vi "Orientation measurements standalone.vi"() -> ()   [LabVIEW 2016]
uses:
  <vilib>/rvi/interface/nirviReadWriteControl/nirviReadWriteControl.xnode
  FPGA Bitfiles/FPGAIMU_FPGATarget_FPGAIMURead_c-b2E2IVPMQ.lvbitx
  <vilib>/rvi/errors/niLvFpgaMergeErrorWithErrorCode.vi
  <vilib>/rvi/errors/niLvFpgaAdjustHostInterfaceError.vi
panel:
  out "Number of misses":i16
  out "Time to read start bit":u32
  out "Time to read data bits":u32
  out "Time to read 1 char":u32
  in  "ThirdTune":u32
  in  "SecondTune":u32=5
  in  "FirstTune":u32
  out "Fifo full?":bool
  in  "Bytes to Read":u32=38
  out "Output":cluster{dbl, dbl, bool}
  out "Error out":errorcluster
  in  "Stop":bool
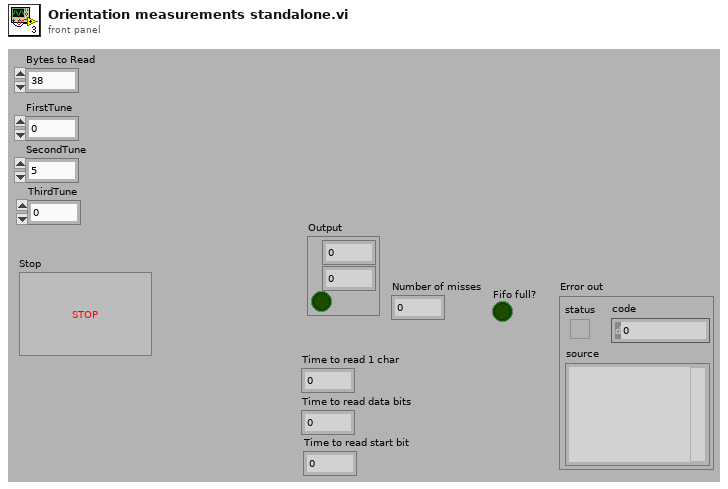
[diagram p1: front panel]
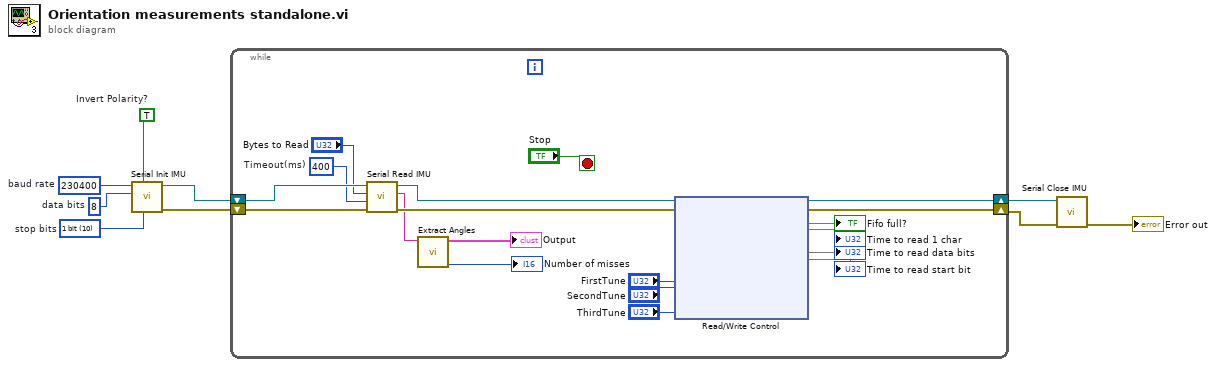
[diagram p0: block diagram]
diagram:
  w9 = u16 10 items=["1 bit"=10, "1.5 bits"=15, "2 bits"=20]  # stop bits
  w8 = 8  # data bits
  w6 = TRUE  # Invert Polarity?
  w7 = u32 230400  # baud rate
  n1 = call "Serial Init IMU.vi"("stop bits (10: 1 bit)"=w9, "Invert Polarity?"=w6, "data bits (8)"=w8, "baud rate (9600)"=w7) -> ("error out"=w2:errorcluster, "FPGA IMU OUT"=w3:refnum<k20>)  [unwired: 6 in]
  n2 = while {
    shift-right: [w26] -> w4
    shift-left: w3 -> [w27]
    shift-right: [w12] -> w1
    shift-left: w2 -> [w17]
    stop <- "Stop" stop-if-true
    w21 = 400  # Timeout(ms)
    n3 = call "Serial Read IMU.vi"("error in (no error)"=w17, "Timeout (ms) (-1: no timeout)"=w21, "Bytes to Read"="Bytes to Read", "FPGA IMU IN"=w27) -> ("error out"=w19:errorcluster, "String"=w13:string, "FPGA IMU OUT"=w18:refnum<k20>)  [unwired: 5 in]
    n4 = call "Extract Angles.vi"("String in"=w13) -> ("Number of misses"=→"Number of misses":i16, "Output"=→"Output":cluster{dbl, dbl, bool})  [unwired: 9 in]
    n5 = xnode "Read/Write Control"("FPGA VI Reference In"=w18, "error in"=w19, "FirstTune"="FirstTune", "SecondTune"="SecondTune", "ThirdTune"="ThirdTune") -> ("FPGA VI Reference Out"=w26:refnum<k20>, "error out"=w12:errorcluster, "Fifo full?"=→"Fifo full?", "Time to read 1 char"=→"Time to read 1 char", "Time to read data bits"=→"Time to read data bits", "Time to read start bit"=→"Time to read start bit")
  }
  n6 = call "Serial Close IMU.vi"("error out"=w1, "FPGA IMU IN 2"=w4) -> ("error out"=→"Error out":errorcluster)  [unwired: 9 in]
